vi "Create.vi"(8 "error in (no error)":errorcluster, 10 "Pattern":string) -> (0 "error out":errorcluster, 3 "String Argument Matching Comparator":refnum<class "String Argument Matching Comparator.lvclass">)   [LabVIEW 2020, in "String Argument Matching Comparator.lvclass"]
uses:
  String Argument Matching Comparator.lvclass
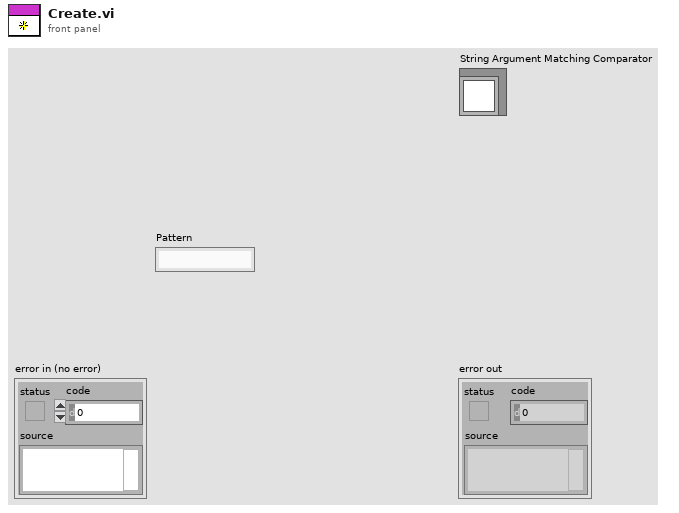
[diagram p1: front panel]
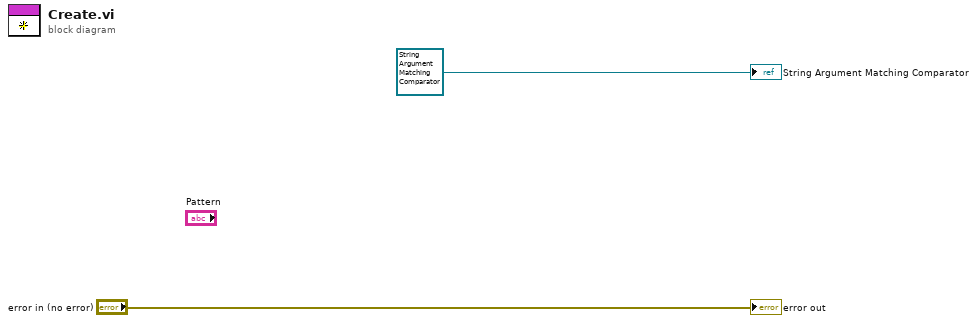
[diagram p0: block diagram]
diagram:
  "error out" <- "error in (no error)"
  "String Argument Matching Comparator" <- refnum<class "String Argument Matching Comparator.lvclass"> refnum ("String Argument Matching Comparator")
